vi "disable_detectors.vi"(8 "error in (no error)":errorcluster, 11 "DL090324Microscope in":refnum<class "InstrumentDL090324.lvclass">) -> (0 "error out":errorcluster, 3 "DL090324Microscope out":refnum<class "InstrumentDL090324.lvclass">)   [LabVIEW 2010, in "InstrumentDL090324.lvclass"]
uses:
  InstrumentDL090324.lvclass
  InstrumentDL090324.lvclass/InstrumentDL090324.ctl
  Detector/GenericDetector/GenericDetector/GenericDetector.lvclass
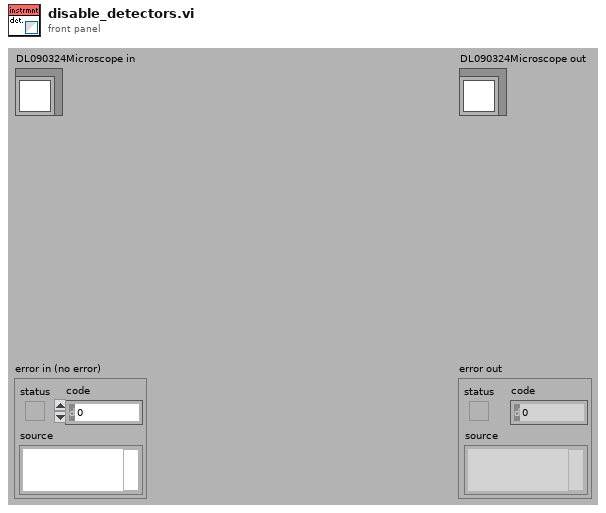
[diagram p1: front panel]
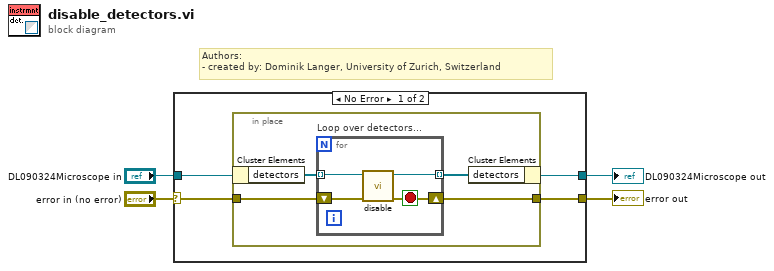
[diagram p0: block diagram]
diagram:
  # "Authors: \n- created by: Dominik Langer, University of Zurich, Switzerland"
  n1 = case shown="No Error" "error in (no error)" {
    selector: "error in (no error)" -> [w8 w18]
    tunnel: [w7 w18] -> w3
    tunnel: [w5 w17] -> w1
    tunnel: "DL090324Microscope in" -> [w6 w17]
    frame No Error {
      n2 = in-place {
        in-place-border: w8 -> [w12]
        in-place-border: [w11] -> w7
        n3 = in-place-cluster #1(w6) -> ("detectors"=w9:refnum<class "GenericDetector.lvclass">[])
        n4 = for "Loop over detectors..." {
          shift-right: [w13] -> w11
          shift-left: w12 -> [w16]
          tunnel: [w15] -> w10 mode=indexing
          tunnel: w9 -> [w14] mode=indexing
          stop <- w13 stop-if-true
          n5 = call-dynamic "disable.vi"("error in (no error)"=w16, "GenericEmissionSensor in"=w14) -> ("error out"=w13:errorcluster, "GenericEmissionSensor out"=w15:refnum<class "GenericDetector.lvclass">)  [unwired: 8 out]
        }
        n6 = in-place-cluster #1("detectors"=w10) -> (w5:refnum<class "InstrumentDL090324.lvclass">)
      }
    }
    frame Error {
    }
  }
  "error out" <- w3
  "DL090324Microscope out" <- w1
